vi "Date.vi"() -> (0 "Current Time":string, 3 "YYYYMMDD Date":string)   [LabVIEW 2017]
panel:
  out "A2":string
  out "A3":string
  out "Current Date":string
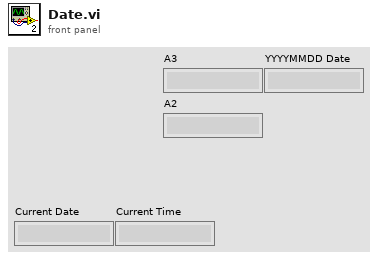
[diagram p1: front panel]
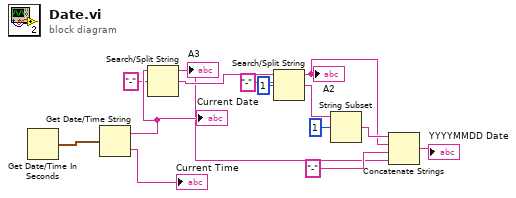
[diagram p0: block diagram]
diagram:
  n1 = Get Date/Time In Seconds() -> (seconds since 1Jan1904=w14:timestamp)
  n2 = Get Date/Time String(seconds (now)=w14) -> (date string=w12:string, time string=→"Current Time":string)  [unwired: 2 in]
  "Current Date" <- w12
  n3 = Search/Split String(string=w12, search string/char (-)="-") -> (substring before match=w3:string, match + rest of string=w10:string)  [unwired: 1 in, 1 out]
  "A3" <- w3
  n4 = Search/Split String(string=w10, search string/char (-)="-", offset (0)=1) -> (substring before match=w5:string, match + rest of string=w8:string)  [unwired: 1 out]
  "A2" <- w5
  n5 = String Subset(string=w8, offset (0)=1) -> (substring=w6:string)  [unwired: 1 in]
  n6 = Concatenate Strings(w6, w5, "-" ("search string/char (-)"), w3) -> (→"YYYYMMDD Date":string)
